vi "Configure DC Input Resistance.vi"(8 "error in (no error)":errorcluster, 10 "DC Input Resistance(0: 10M)":u16(ring) items=["10M", ">10G"], 11 "VISA resource name":refnum<visa-resource-name>) -> (0 "error out":errorcluster, 3 "VISA resource name out":refnum<visa-resource-name>)   [LabVIEW 2020, in "Library Instrument & Equipement.lvlib" / "Library Multimeter.lvlib" / "RIGOL DM3058.lvlib"]
doc: "Configures the DC Input Resistance."
uses:
  RIGOL DM3058.lvlib
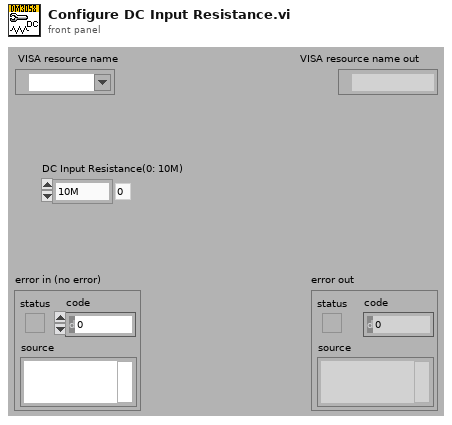
[diagram p1: front panel]
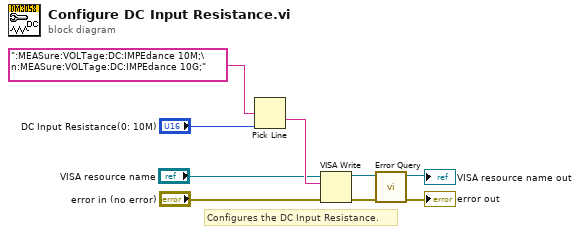
[diagram p0: block diagram]
diagram:
  # "Configures the DC Input Resistance."
  n1 = Pick Line(multi-line string=":MEASure:VOLTage:DC:IMPEdance 10M;\n:MEASure:VOLTage:DC:IMPEdance 10G;", line index="DC Input Resistance(0: 10M)") -> (output string=w7:string)  [unwired: 1 out]
  n2 = VISA Write(VISA resource name="VISA resource name", write buffer=w7, error in (no error)="error in (no error)") -> (VISA resource name out=w4:refnum<visa-resource-name>, error out=w3:errorcluster)  [unwired: 1 out]
  n3 = call "Error Query.vi"("error in (no error)"=w3, "VISA resource name"=w4) -> ("error out"=→"error out":errorcluster, "VISA resource name out"=→"VISA resource name out":refnum<visa-resource-name>)  [unwired: 6 in, 2 out]
